vi "Callback Change Direction.vi"(6 "Variant":variant, 8 "error in (no error)":errorcluster, 9 "Old Values":string[][](array[string]), 10 "object ref in":T2, 11 "Table Change":T3) -> (0 "error out":errorcluster)   [LabVIEW 2013, in "shared memory editor node.lvclass"]
doc: "This VI gets called automatically when changes are made to the 'Channel Direction' column of the table and must handle changes appropriately. Register this callback using the appropriate 'Define Column' VI from the Table API."
uses:
  shared memory editor node.lvclass
  <vilib>/NI/DCAF/Tag Editor Core/Table API/Table Manager/Cell Change.ctl
  <vilib>/NI/DCAF/Tag Editor Core/Table API/Table Manager/object ref.ctl
  <vilib>/NI/DCAF/Tag Editor Core/Configuration Editor/Classes/Engine Parent/Engine Parent Editor Node.lvclass
  <vilib>/NI/DCAF/Tag Editor Core/Configuration Editor/Classes/Module editor node/module editor node.lvclass
  Permissions Enum.ctl
  module/configuration/shared memory configuration.lvclass
  module/configuration/shared memory configuration.lvclass/shared memory configuration.ctl
  <vilib>/NI/Tag Bus Module Framework/channel/TBM channel.lvclass/TBM channel.ctl
  <vilib>/NI/Configuration Framework/serializable configuration/NISE_CEF_serializable configuration.lvclass/NISE_CEF_serializable configuration.ctl
  <vilib>/Utility/LVClass/Get LV Class Name.vi
  <vilib>/NI/Configuration Framework/error generator/NISE_error generator.vi
  <vilib>/NI/DCAF/Tag Editor Core/Table API/Table Manager.lvlib
  <vilib>/NI/Tag Bus Module Framework/channel/TBM channel.lvclass
  <vilib>/NI/Configuration Framework/serializable configuration/NISE_CEF_serializable configuration.lvclass
  <vilib>/NI/Module Execution Interface/Engine Configuration/engine configuration.lvclass
  <vilib>/NI/DCAF/Tag Editor Core/Table API/Table Manager/Table Manager.lvclass
panel:
  in  "Permissions":T1
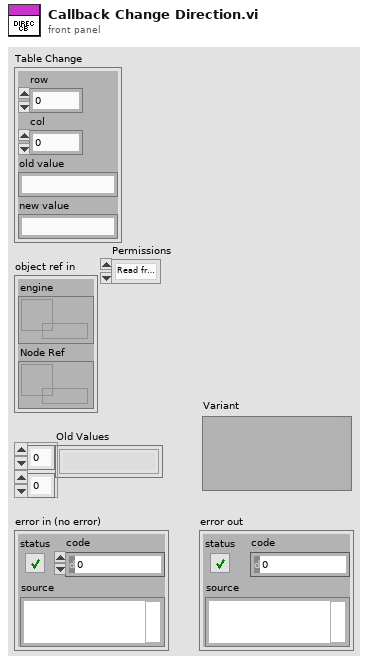
[diagram p1: front panel]
types:
  T1 = typedef "shared memory editor node.lvclass/Permissions Enum.ctl" = enum16{"Read from HW", "Write to HW"}
  T2 = typedef "Table Manager.lvlib/Table Manager.lvclass/object ref.ctl" = cluster{"engine":refnum<data-value>, "Node Ref":refnum<data-value>}
  T3 = typedef "Table Manager.lvlib/Cell Change.ctl" = cluster{"row":i32, "col":i32, "old value":string, "new value":string}
  T4 = typedef "TBM channel.lvclass/channel classification.ctl" = enum16{"input data", "output data", "processing parameter", "processing result"}
  T5 = typedef "shared memory configuration.lvclass/Line.ctl" = cluster{"channel":refnum<class "TBM channel.lvclass">}
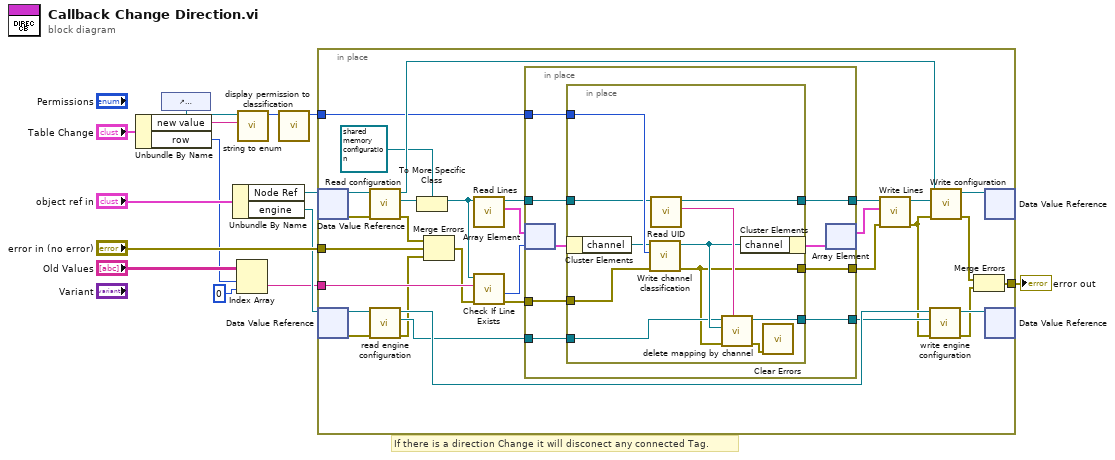
[diagram p0: block diagram]
diagram:
  # "If there is a direction Change it will disconect any connected Tag."
  n1 = Unbundle By Name("Table Change") -> ("new value"=w1:string, "row"=w2:i32)
  n2 = control-ref of="Permissions"() -> (w8:refnum<vi>)
  n3 = Unbundle By Name("object ref in") -> ("Node Ref"=w11:refnum<data-value>, "engine"=w10:refnum<data-value>)
  n4 = Index Array(array="Old Values", index (row)=w2, index (col)=0 ("disabled index (col)")) -> (element=w3:string)
  n5 = call <vilib>:"string to enum.vi"("String"=w1, "Enum"=w8) -> ("Value"=w7:i32)  [unwired: 8 in, 1 out]
  n6 = call "display permission to classification.vi"("display permissions"=w7) -> ("channel classification"=w6:T4)  [unwired: 10 in]
  n7 = in-place {
    in-place-border: [w38] -> w14
    in-place-border: "error in (no error)" -> [w16]
    in-place-border: w6 -> [w26]
    in-place-border: w3 -> [w25]
    n8 = in-place-dvr #1(w11) -> (w35:refnum<class "module editor node.lvclass">, w37:errorcluster)
    n9 = in-place-dvr #2(w10) -> (w44:refnum<class "Engine Parent Editor Node.lvclass">, w45:errorcluster)
    n10 = call-dynamic "Read configuration.vi"("error in"=w37, "NISE_CEF_serializable node in"=w35) -> ("error out"=w36:errorcluster, "configuration"=w33:refnum<class "NISE_CEF_serializable configuration.lvclass">, "NISE_CEF_serializable node out"=w34:refnum<class "module editor node.lvclass">)  [unwired: 7 in]
    n11 = call <vilib>:"read engine configuration.vi"("error in"=w45, "Engine Parent Editor Node in"=w44) -> ("error out"=w15:errorcluster, "engine configuration"=w22:refnum<class "engine configuration.lvclass">, "Engine Parent Editor Node out"=w41:refnum<class "Engine Parent Editor Node.lvclass">)  [unwired: 7 in]
    n12 = To More Specific Class(target class=refnum<class "shared memory configuration.lvclass"> refnum ("tag bus configurable plugin module configuration"), reference=w33) -> (specific class reference=w30:refnum<class "shared memory configuration.lvclass">)  [unwired: 1 in, 1 out]
    n13 = Merge Errors(w36, w16, w15) -> (w20:errorcluster)
    n14 = call "Read Lines.vi"("shared memory configuration in"=w30) -> ("Lines"=w29:T5[], "shared memory configuration out"=w24:refnum<class "shared memory configuration.lvclass">)  [unwired: 8 in, 1 out]
    n15 = call-dynamic "Check If Line Exists.vi"("error in"=w20, "Name to Locate"=w25, "shared memory configuration in"=w30) -> ("error out"=w19:errorcluster, "Index"=w27:i32)  [unwired: 4 in, 3 out]
    n16 = in-place {
      in-place-border: w26 -> [w52]
      in-place-border: w24 -> [w51]
      in-place-border: [w50] -> w23
      in-place-border: w22 -> [w49]
      in-place-border: [w48] -> w21
      in-place-border: w19 -> [w47]
      in-place-border: [w46] -> w18
      n17 = in-place-array #3(w29, w27) -> (w54:T5)
      n18 = in-place {
        in-place-border: w52 -> [w65]
        in-place-border: w51 -> [w64]
        in-place-border: [w63] -> w50
        in-place-border: w49 -> [w57]
        in-place-border: [w61] -> w48
        in-place-border: w47 -> [w58]
        in-place-border: [w55] -> w46
        n19 = in-place-cluster #4(w54) -> ("channel"=w62:refnum<class "TBM channel.lvclass">)
        n20 = call <vilib>:"Write channel classification.vi"("error in"=w58, "channel classification"=w65, "channel in"=w62) -> ("error out"=w55:errorcluster, "channel out"=w59:refnum<class "TBM channel.lvclass">)  [unwired: 7 in]
        n21 = call <vilib>:"Read UID.vi"("configuration in"=w64) -> ("instance id"=w60:string, "configuration out"=w63:refnum<class "shared memory configuration.lvclass">)  [unwired: 8 in, 1 out]
        n22 = call <vilib>:"delete mapping by channel.vi"("owner ID"=w60, "error in"=w55, "channel"=w59, "engine configuration in"=w57) -> ("error out"=w56:errorcluster, "engine configuration out"=w61:refnum<class "engine configuration.lvclass">)  [unwired: 6 in]
        n23 = in-place-cluster #4("channel"=w59) -> (w53:T5)
        n24 = call <vilib>:"Clear Errors.vi"("error in (no error)"=w56) -> ()  [unwired: 6 in, 1 out]
      }
      n25 = in-place-array #3(w53) -> (w28:T5[])  [unwired: 1 out]
    }
    n26 = call "Write Lines.vi"("error in (no error)"=w18, "Lines"=w28, "shared memory configuration in"=w23) -> ("error out"=w17:errorcluster, "shared memory configuration out"=w31:refnum<class "shared memory configuration.lvclass">)  [unwired: 7 in]
    n27 = call <vilib>:"write engine configuration.vi"("error in"=w17, "engine configuration"=w21, "Engine Parent Editor Node in"=w41) -> ("error out"=w40:errorcluster, "Engine Parent Editor Node out"=w43:refnum<class "Engine Parent Editor Node.lvclass">)  [unwired: 7 in]
    n28 = call-dynamic "Write configuration.vi"("error in"=w17, "configuration"=w31, "NISE_CEF_serializable node in"=w34) -> ("error out"=w39:errorcluster, "NISE_CEF_serializable node out"=w42:refnum<class "module editor node.lvclass">)  [unwired: 7 in]
    n29 = Merge Errors(w39, w40) -> (w38:errorcluster)
    n30 = in-place-dvr #1(w42) -> ()  [unwired: 2 out]
    n31 = in-place-dvr #2(w43) -> ()  [unwired: 2 out]
  }
  "error out" <- w14
